vi "Set path.vi"(8 "error in":errorcluster, 10 "Path set?":bool, 11 "Path in":path) -> (0 "error out":errorcluster, 2 "cancelled?":bool, 3 "Path out":path)   [LabVIEW 2020]
uses:
  <vilib>/Utility/sysdir.llb/System Directory Type.ctl
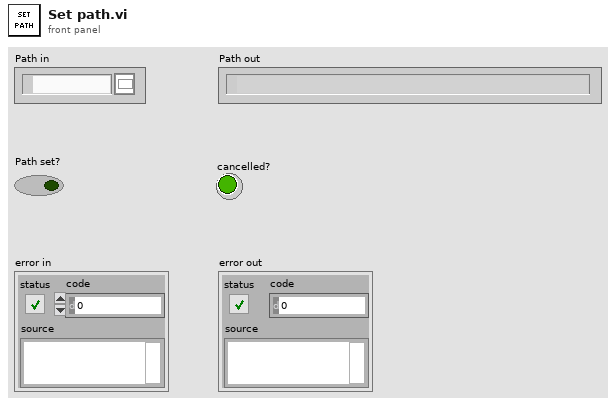
[diagram p1: front panel]
types:
  T1 = typedef "System Directory Type.ctl" = i32
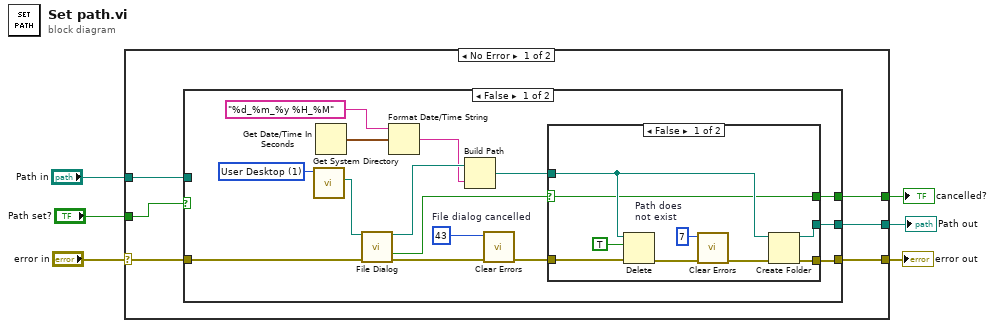
[diagram p0: block diagram]
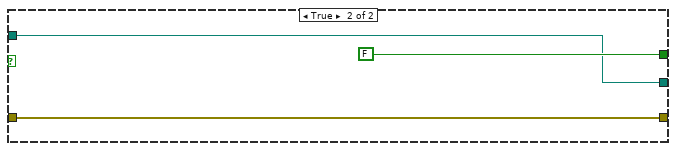
[diagram p3: hidden frame]
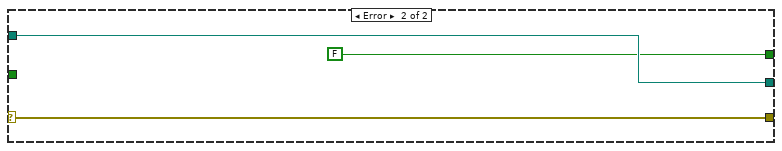
[diagram p4: hidden frame]
diagram:
  n1 = case shown="No Error" "error in" {
    selector: "error in" -> [w9 w44]
    tunnel: "Path in" -> [w12 w43]
    tunnel: [w11 FALSE ("cancelled")] -> w5
    tunnel: [w10 w43] -> w4
    tunnel: "Path set?" -> [w8 _]
    tunnel: [w7 w44] -> w1
    frame No Error {
      n2 = case shown="False" w8 {
        tunnel: w9 -> [w25 w39]
        tunnel: [w17 w40] -> w10
        tunnel: [w13 FALSE ("cancelled")] -> w11
        tunnel: w12 -> [_ w40]
        tunnel: [w18 w39] -> w7
        frame False {
          w23 = 43  # File dialog cancelled
          w26 = T1 1 items=["User Home"=0, "User Desktop"=1, "User Documents"=2, "User Application Data"=3, "User Preferences"=4, "User Temporary"=5, "Public Documents"=6, "Public Application Data"=7, "Public Preferences"=8, "Public Cache"=13, "System Core Libraries"=9, "System Installed Libraries"=10, "Application Files"=11, "Boot Volume Root"=12] ("system directory type")
          n3 = call <vilib>:"Get System Directory.vi"("system directory type"=w26) -> ("system directory"=w27:path)  [unwired: 10 in]
          n4 = Get Date/Time In Seconds() -> (seconds since 1Jan1904=w22:timestamp)
          n5 = call "File Dialog"("start path"=w27, "error in"=w25) -> ("selected path"=w20:path, "cancelled"=w14:bool, "error out"=w24:errorcluster)  [unwired: 10 in, 1 out]
          n6 = Format Date/Time String(time format string (%c)="%d_%m_%y %H_%M", seconds (now)=w22) -> (date/time string=w19:string)  [unwired: 1 in]
          n7 = Build Path(base path=w20, name or relative path=w19) -> (appended path=w15:path)
          n8 = call <vilib>:"Clear Errors.vi"("error in (no error)"=w24, "specific error code to clear (0: all)"=w23) -> ("error out"=w16:errorcluster)  [unwired: 4 in, 1 out]
          n9 = case shown="False" w14 {
            selector: w14 -> [w28 w38]
            tunnel: [w36 w37] -> w18
            tunnel: [w35 _] -> w17
            tunnel: w16 -> [w34 w37]
            tunnel: w15 -> [w33 _]
            tunnel: [w28 w38] -> w13
            frame False {
              w29 = 7  # Path does not exist
              n10 = Delete(path (use dialog)=w33, entire hierarchy (F)=TRUE, error in=w34) -> (error out=w31:errorcluster)  [unwired: 2 in, 2 out]
              n11 = call <vilib>:"Clear Errors.vi"("error in (no error)"=w31, "specific error code to clear (0: all)"=w29) -> ("error out"=w30:errorcluster)  [unwired: 4 in, 1 out]
              n12 = Create Folder(path (use dialog)=w33, error in=w30) -> (created path=w35:path, error out=w36:errorcluster)  [unwired: 1 in, 1 out]
            }
            frame True {
            }
          }
        }
        frame True {
        }
      }
    }
    frame Error {
    }
  }
  "Path out" <- w4
  "cancelled?" <- w5
  "error out" <- w1
